vi "Build Path.vi"(6 "Unique ID":string, 7 "Parent ID":string, 10 "Parent Definition":refnum<class "Linked List Definition.lvclass">, 11 "Linked List Definition in":refnum<class "Linked List Definition.lvclass">) -> (2 "Path":string, 3 "Linked List Definition out":refnum<class "Linked List Definition.lvclass">)   [LabVIEW 2020, in "Linked Lists.lvlib" / "Linked List Definition.lvclass"]
uses:
  <vilib>/gpm_packages/@cs/linked-list/Source/Linked List/Linked List Definition/Linked List Definition.lvclass
  <vilib>/gpm_packages/@cs/linked-list/Source/Linked List/Linked List Definition/Linked List Definition.lvclass/Linked List Definition.ctl
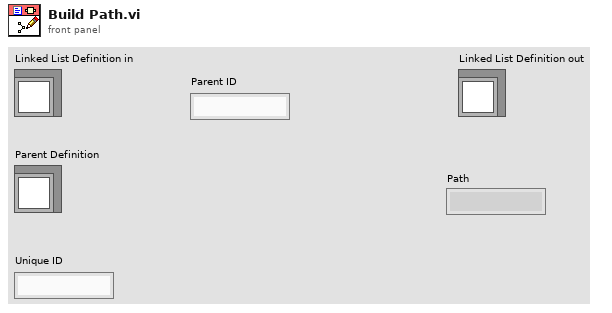
[diagram p1: front panel]
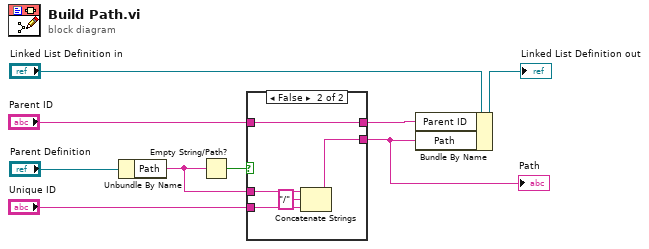
[diagram p0: block diagram]
diagram:
  n1 = Unbundle By Name("Parent Definition") -> ("Path"=w6:string)
  n2 = Empty String/Path?(string/path=w6) -> (empty?=w8:bool)
  n3 = case shown="False" w8 {
    tunnel: w6 -> [_ w16]
    tunnel: [w11 w14] -> w3
    tunnel: "Unique ID" -> [w11 w13]
    tunnel: [w10 w12] -> w4
    tunnel: "Parent ID" -> [w10 w12]
    frame True {
    }
    frame False {
      n4 = Concatenate Strings(w16, "/" ("string"), w13) -> (w14:string)
    }
  }
  "Path" <- w3
  n5 = Bundle By Name(cluster="Linked List Definition in", "Parent ID"=w4, "Path"=w3) -> (→"Linked List Definition out":refnum<class "Linked List Definition.lvclass">)
